vi "Fetch Power Measurement Statistics Trace.vi"(8 "error in (no error)":errorcluster, 9 "Result Type (Amplitude Probability Density)":i32(ring) items=["Amplitude Probability Density", "Complementary Cumulative Distribution Function"], 10 "Instance (1)":i32=1, 11 "VISA resource name":refnum<visa-resource-name>) -> (0 "error out":errorcluster, 1 "Results":dbl[](array[numeric]) format="%^.3e", 2 "Reliability":i32, 3 "VISA resource name out":refnum<visa-resource-name>)   [LabVIEW 2020, in "Rohde&Schwarz CMXP GPRF.lvlib"]
doc: "Returns the trace points of the complementary cumulative distribution VI or the amplitude probability density.\nThis result is only available in \"Statistic\" evaluation mode (rscmwgprf Configure Power Measurement Result Mode.vi).\n\nAttributes:\nRSCMXPGPRF_ATTR_FETCH_POWER_MEASUREMENT_STATISTICS_TRACE_APD\nRSCMXPGPRF_ATTR_FETCH_POWER_MEASUREMENT_STATISTICS_TRACE_CCDF\n\nRemote-control commands:\nFETCh:GPRF:MEAS<i>:POWer:APD?\nFETCh:GPRF:MEAS<i>:POWer:CCDF?"
uses:
  <instrlib>/Rohde&Schwarz CMXP GPRF/Rohde&Schwarz CMXP GPRF.lvlib
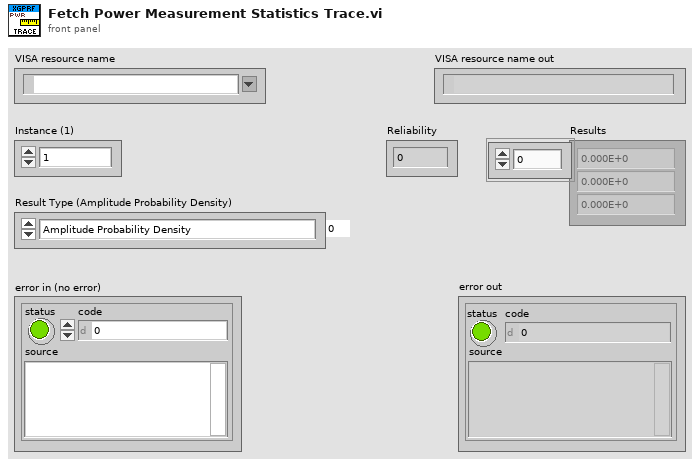
[diagram p1: front panel]
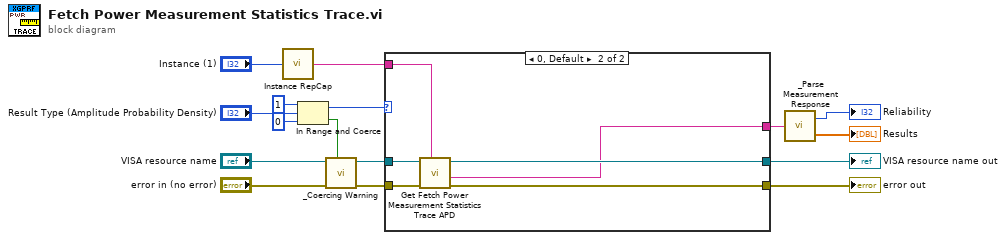
[diagram p0: block diagram]
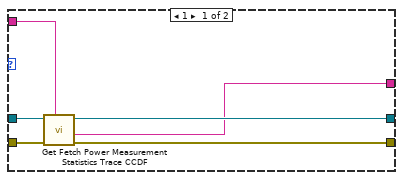
[diagram p2: hidden frame]
diagram:
  n1 = call <instrlib>:"Instance RepCap.vi"("Instance in"="Instance (1)") -> ("Instance out"=w5:string)
  n2 = In Range and Coerce(upper limit=1, x="Result Type (Amplitude Probability Density)", lower limit=0) -> (coerced(x)=w4:i32, In Range?=w7:bool)
  n3 = call <instrlib>:"_Coercing Warning.vi"("In Range?"=w7, "error in (no error)"="error in (no error)", "VISA resource name"="VISA resource name") -> ("error out"=w11:errorcluster, "VISA resource name out"=w10:refnum<visa-resource-name>)  [unwired: 7 in]
  n4 = case shown="0, Default" w4 {
    tunnel: w11 -> [w22 w28]
    tunnel: w10 -> [w21 w27]
    tunnel: [w20 w26] -> w9
    tunnel: [w19 w25] -> w8
    tunnel: w5 -> [w18 w24]
    tunnel: [w17 w23] -> w3
    frame 1 {
      n5 = call "Get Fetch Power Measurement Statistics Trace CCDF"("Repeated Capabilities"=w18, "error in (no error)"=w22, "instrument handle"=w21) -> ("error out"=w20:errorcluster, "Fetch Power Measurement Statistics Trace CCDF"=w17:string, "instrument handle out"=w19:refnum<visa-resource-name>)  [unwired: 6 in]
    }
    frame 0, Default {
      n6 = call "Get Fetch Power Measurement Statistics Trace APD"("Repeated Capabilities"=w24, "error in (no error)"=w28, "instrument handle"=w27) -> ("error out"=w26:errorcluster, "Fetch Power Measurement Statistics Trace APD"=w23:string, "instrument handle out"=w25:refnum<visa-resource-name>)  [unwired: 6 in]
    }
  }
  "error out" <- w9
  "VISA resource name out" <- w8
  n7 = call <instrlib>:"_Parse Measurement Response.vi"("String In"=w3) -> ("Reliability"=→"Reliability":i32, "Data"=→"Results":dbl[])
